vi "Start Tracing (Capture to File).vi"(8 "error in (no error)":errorcluster, 10 "file write mode (create)":T1(ring), 11 "log file path":path) -> (0 "error out":errorcluster)   [LabVIEW 2011, in "NI IO Trace.lvlib"]
doc: "Commands NI I/O Trace to start logging to a file. The type of file is dependent on the extension of the file path passed to the VI. Valid file types are .nitrace, .txt, and .csv. Trace files (.nitrace) contain the most information and are recommended for all applications not requiring parsing by an external program."
uses:
  <vilib>/NiIOTrace/NI IO Trace.lvlib
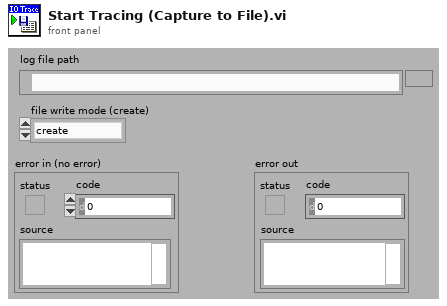
[diagram p1: front panel]
types:
  T1 = enum32{"create", "append or create", "replace or create"}
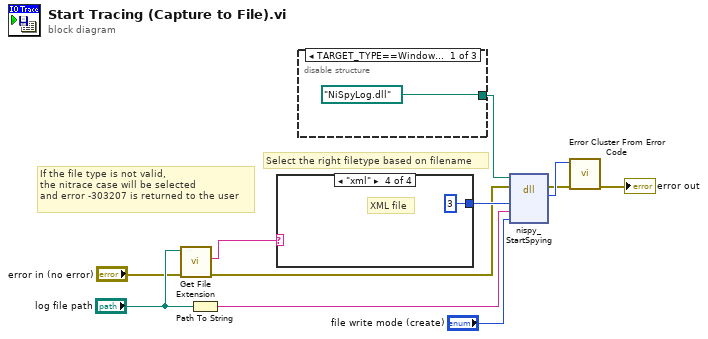
[diagram p0: block diagram]
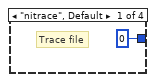
[diagram p2: hidden frame]
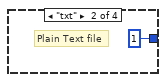
[diagram p3: hidden frame]
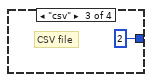
[diagram p4: hidden frame]
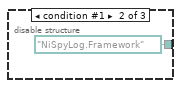
[diagram p5: hidden frame]
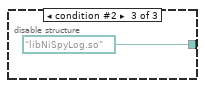
[diagram p6: hidden frame]
diagram:
  # "If the file type is not valid,\nthe nitrace case will be selected\nand error -303207 is returned to the user"
  # "Select the right filetype based on filename"
  n1 = call <vilib>:"Get File Extension.vi"("error in (no error)"="error in (no error)", "file"="log file path") -> ("error out"=w1:errorcluster, "lowercase file extension"=w5:string)  [unwired: 8 out]
  n2 = Path To String(path="log file path") -> (string=w7:string)
  n3 = case shown="\"xml\"" w5 {
    tunnel: [0 ("log file format (do not log to file)") 1 ("log file format (do not log to file)") 2 ("log file format (do not log to file)") 3 ("log file format (do not log to file)")] -> w4
    frame "nitrace", Default {
      # "Trace file"
    }
    frame "txt" {
      # "Plain Text file"
    }
    frame "csv" {
      # "CSV file"
    }
    frame "xml" {
      # "XML file"
    }
  }
  n4 = disable-structure shown="TARGET_TYPE==Windows, default" {
    disable-tunnel: [path "NiSpyLog.dll" ("path in") path "NiSpyLog.Framework" ("path in") path "libNiSpyLog.so" ("path in")] -> w10
    frame condition #0 (active) {
    }
    frame condition #1 {
    }
    frame condition #2 {
    }
  }
  n5 = dll-call lib="C:/WINDOWS/system32/NiSpyLog.dll" fn="nispy_StartSpying"(path in=w10, error in=w1, "logFileSetting"=w4, "filePathString"=w7, "overwriteFile"="file write mode (create)") -> (error out=w9:errorcluster, "return type"=w11:i32)  [unwired: 3 in, 2 out]
  n6 = call <vilib>:"Error Cluster From Error Code.vi"("error in (no error)"=w9, "error code (0)"=w11) -> ("error out"=→"error out":errorcluster)  [unwired: 1 in, 6 out]
